vi "Get Legend Display.vi"(6 "Control Ref Queue":T1, 8 "error in (no error)":errorcluster, 9 "Auto Size?":bool, 11 "Legend Cluster":T2(array[cluster])) -> (0 "error out":errorcluster)   [LabVIEW 2017, in "2D Plot.lvclass"]
uses:
  <vilib>/Math Plots/2D Math Plots/2D Plot/2D Plot/2D Plot.lvclass
  <vilib>/Math Plots/2D Math Plots/2D Plot/Action String/2DMathPlot Ctrl Act Queue.ctl
  <vilib>/Math Plots/2D Math Plots/2D Plot/Action String/2DMathPlot Ctrl Act Cluster.ctl
  <vilib>/Math Plots/2D Math Plots/2D Plot/Action String/2DMathPlot State Class.ctl
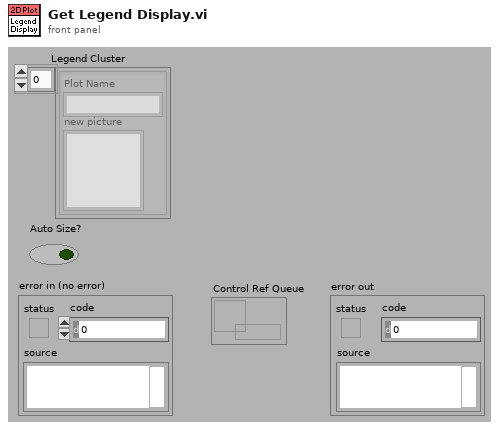
[diagram p1: front panel]
types:
  T1 = typedef "2DMathPlot Ctrl Act Queue.ctl" = refnum<queue>
  T2 = cluster{"Plot Name":string, "new picture":picture}[]
  T3 = enum16{"User-specified Font", "Application Font", "System Font", "Dialog Font"}
  T4 = typedef "2DMathPlot Ctrl Act Cluster.ctl" = cluster{"Plot Area Ref":refnum<vi>, "Z Axis Ref":refnum<vi>, "Legend Ref":refnum<vi>, "XControl Ref":refnum<vi>, "Facade Ref":refnum<vi>, "Display State Change Class":T5}
  T5 = typedef "2DMathPlot State Class.ctl" = enum16{"Update All (Undo)", "Update General", "Update Appearance", "Update Format", "Update Scale", "Update Marker", "Update Cursor", "None"}
  T6 = cluster{"left":i16, "top":i16, "right":i16, "bottom":i16}
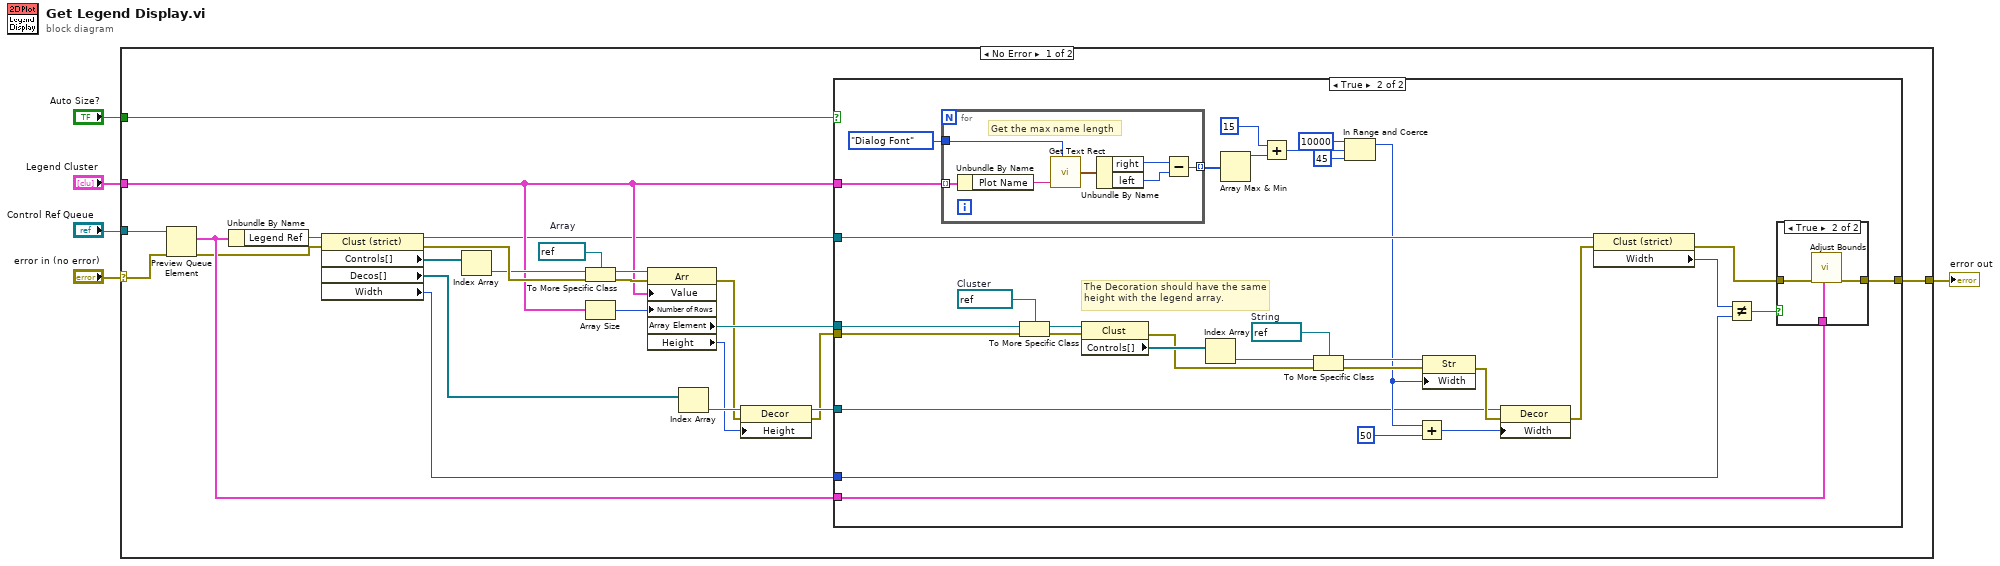
[diagram p0: block diagram]
diagram:
  n1 = case shown="No Error" "error in (no error)" {
    selector: "error in (no error)" -> [w15 w74]
    tunnel: "Control Ref Queue" -> [w17 _]
    tunnel: [w28 w74] -> w5
    tunnel: "Legend Cluster" -> [w20 _]
    tunnel: "Auto Size?" -> [w12 _]
    frame No Error {
      w23 = refnum<vi> refnum  # Array
      n2 = Preview Queue Element(queue=w17, error in (no error)=w15) -> (element=w16:T4, error out=w14:errorcluster)  [unwired: 3 out]
      n3 = Unbundle By Name(w16) -> ("Legend Ref"=w29:refnum<vi>)
      n4 = property class="Clust (strict)"(reference=w29, error in=w14) -> (reference out=w19:refnum<vi>, error out=w27:errorcluster, "Controls[]"=w21:refnum<vi>[], "Decos[]"=w11:refnum<vi>[], "Width"=w18:u32)
      n5 = Index Array(array=w21) -> (element=w22:refnum<vi>)  [unwired: 1 in]
      n6 = To More Specific Class(target class=w23, reference=w22, error in=w27) -> (specific class reference=w25:refnum<vi>, error out=w24:errorcluster)
      n7 = Array Size(array=w20) -> (size(s)=w13:i32)
      n8 = property class="Arr"(reference=w25, error in=w24, "Value"=w20, "Number of Rows"=w13) -> (error out=w7:errorcluster, "Array Element"=w26:refnum<vi>, "Height"=w8:u32)  [unwired: 1 out]
      n9 = Index Array(array=w11) -> (element=w10:refnum<vi>)  [unwired: 1 in]
      n10 = property class="Decor"(reference=w10, error in=w7, "Height"=w8) -> (reference out=w9:refnum<vi>, error out=w6:errorcluster)
      n11 = case shown="True" w12 {
        tunnel: [w30 w62] -> w28
        tunnel: w6 -> [w30 w58]
        tunnel: w26 -> [_ w50]
        tunnel: w9 -> [_ w31]
        tunnel: w20 -> [_ w48]
        tunnel: w19 -> [_ w47]
        tunnel: w18 -> [_ w45]
        tunnel: w16 -> [_ w41]
        frame False {
        }
        frame True {
          w55 = refnum<vi> refnum  # String
          w51 = refnum<vi> refnum  # Cluster
          # "The Decoration should have the same height with the legend array."
          n12 = for {
            tunnel: w48 -> [w73] mode=indexing
            tunnel: [w68] -> w49 mode=indexing
            tunnel: T3."Dialog Font" ("desired font(Application)") -> [w67]
            # "Get the max name length"
            n13 = Unbundle By Name(w73) -> ("Plot Name"=w69:string)
            n14 = call <vilib>:"Get Text Rect.vi"("desired font(Application)"=w67, "text"=w69) -> ("rect"=w72:T6)  [unwired: 4 in, 3 out]
            n15 = Unbundle By Name(w72) -> ("right"=w71:i16, "left"=w70:i16)
            n16 = Subtract(x=w71, y=w70) -> (x-y=w68:i16)
          }
          n17 = To More Specific Class(target class=w51, reference=w50, error in=w58) -> (specific class reference=w52:refnum<vi>, error out=w59:errorcluster)
          n18 = property class="Clust"(reference=w52, error in=w59) -> (error out=w38:errorcluster, "Controls[]"=w53:refnum<vi>[])  [unwired: 1 out]
          n19 = Index Array(array=w53) -> (element=w56:refnum<vi>)  [unwired: 1 in]
          n20 = Array Max & Min(array=w49) -> (max value=w39:i16)  [unwired: 3 out]
          n21 = Add(x=u32 15 ("y"), y=w39) -> (x+y=w37:u32)
          n22 = To More Specific Class(target class=w55, reference=w56, error in=w38) -> (specific class reference=w54:refnum<vi>, error out=w61:errorcluster)
          n23 = In Range and Coerce(upper limit=u32 10000, x=w37, lower limit=u32 45) -> (coerced(x)=w33:u32)  [unwired: 1 out]
          n24 = Add(x=w33, y=u32 50) -> (x+y=w32:u32)
          n25 = property class="Str"(reference=w54, error in=w61, "Width"=w33) -> (error out=w60:errorcluster)  [unwired: 1 out]
          n26 = property class="Decor"(reference=w31, error in=w60, "Width"=w32) -> (error out=w43:errorcluster)  [unwired: 1 out]
          n27 = property class="Clust (strict)"(reference=w47, error in=w43) -> (error out=w42:errorcluster, "Width"=w46:u32)  [unwired: 1 out]
          n28 = Not Equal?(x=w46, y=w45) -> (x != y?=w44:bool)
          n29 = case shown="True" w44 {
            tunnel: [w63 w65] -> w62
            tunnel: w41 -> [_ w64]
            tunnel: w42 -> [w63 w66]
            frame False {
            }
            frame True {
              n30 = call <vilib>:"Adjust Bounds.vi"("Control Ref Cluster"=w64, "error in (no error)"=w66) -> ("error out"=w65:errorcluster)  [unwired: 9 out]
            }
          }
        }
      }
    }
    frame Error {
    }
  }
  "error out" <- w5
